vi "Core Import Validation.vi"(6 "Slot Number":u32, 7 "File to Import":path, 8 "error in (no error)":errorcluster, 9 "Endpoint Configurations":T1[](array[typedef]), 10 "Switch Properties":T3, 11 "SLSC Switch Import Unit Tests in":refnum<class "SLSC Switch Import Unit Tests.lvclass">) -> (0 "error out":errorcluster, 3 "SLSC Switch Import Unit Tests out":refnum<class "SLSC Switch Import Unit Tests.lvclass">)   [LabVIEW 2017, in "SLSC Switch Import Unit Tests.lvclass"]
uses:
  SLSC Switch Import Unit Tests.lvclass
  Scripting/Properties/SLSC Switch All Properties.ctl
  Shared/Endpoint Configuration Cluster.ctl
  Shared/Endpoint Configuration Enum.ctl
  SLSC Switch Import Unit Tests.lvclass/SLSC Switch Import Unit Tests.ctl
  <userlib>/_OpenG.lib/file/file.llb/Append Path to Root if Relative - Scalar__ogtk.vi
  <vilib>/NI Veristand/Custom Device API/Get Item Property (I32).vi
  Scripting/SLSC Switch Scripting.lvlib
  niveristand-custom-device-testing-tools/VeriStandTestUtilities/VeriStandTestUtilities.lvlib
  <vilib>/NI VeriStand/Custom Device API/Custom Device API.lvlib
  Shared/Routing and Faulting Hardware API/Routing and Faulting Hardware API.lvlib
  Shared/SLSC Switch Shared.lvlib
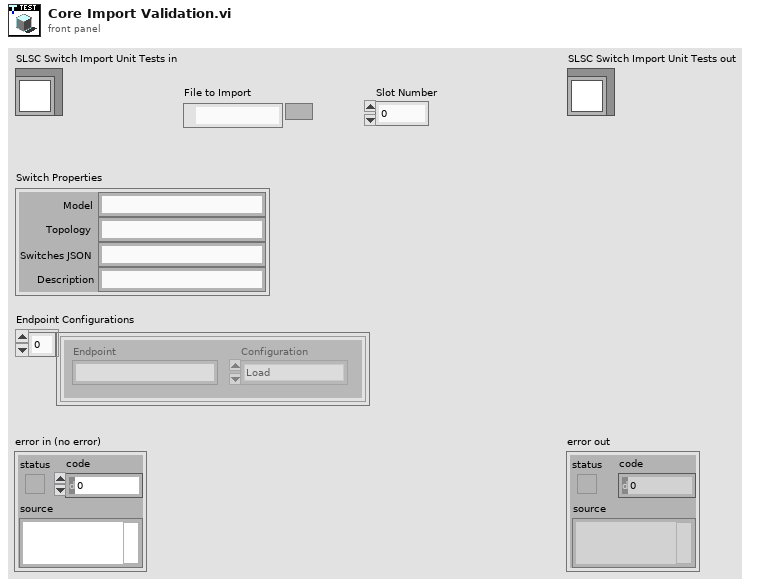
[diagram p1: front panel]
types:
  T1 = typedef "SLSC Switch Shared.lvlib/Endpoint Configuration Cluster.ctl" = cluster{"Endpoint":string, "Configuration":T2}
  T2 = typedef "SLSC Switch Shared.lvlib/Endpoint Configuration Enum.ctl" = enum16{"Load", "Source", "Configuration"}
  T3 = typedef "SLSC Switch Scripting.lvlib/SLSC Switch All Properties.ctl" = cluster{"Model":string, "Topology":string, "Switches JSON":string, "Description":string}
  T4 = typedef "Custom Device API.lvlib/Custom Device Item Ref.ctl" = u64
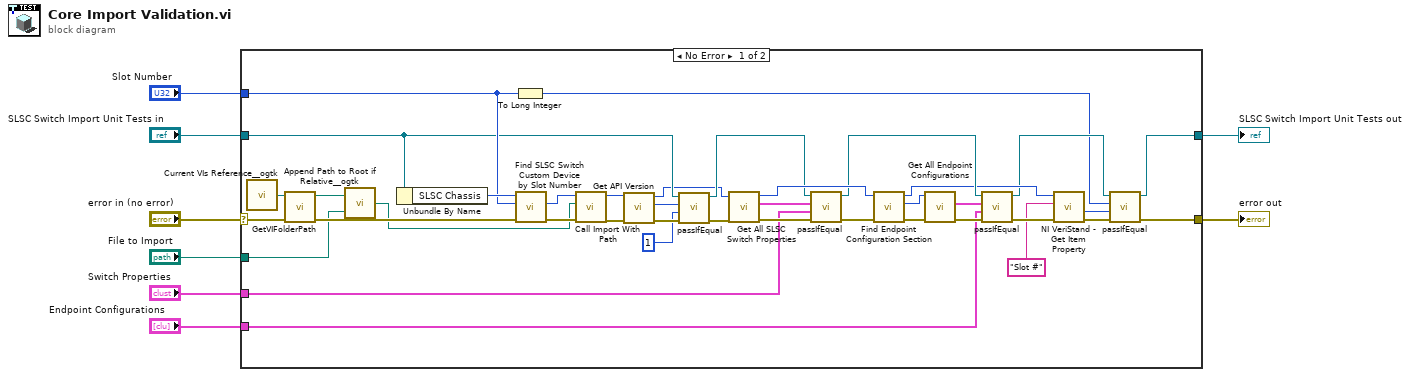
[diagram p0: block diagram]
diagram:
  n1 = case shown="No Error" "error in (no error)" {
    selector: "error in (no error)" -> [w19 w49]
    tunnel: [w18 w49] -> w7
    tunnel: [w20 w48] -> w5
    tunnel: "SLSC Switch Import Unit Tests in" -> [w11 w48]
    tunnel: "File to Import" -> [w24 _]
    tunnel: "Slot Number" -> [w23 _]
    tunnel: "Switch Properties" -> [w22 _]
    tunnel: "Endpoint Configurations" -> [w21 _]
    frame No Error {
      n2 = call <userlib>:"Current VIs Reference__ogtk.vi"() -> ("Current VI's reference"=w44:refnum<vi>)  [unwired: 5 in]
      n3 = call "GetVIFolderPath.vi"("error in (no error)"=w19, "VI Reference in"=w44) -> ("error out"=w42:errorcluster, "VI Folder Path out"=w43:path)  [unwired: 8 in]
      n4 = call-poly <userlib>:"Append Path to Root if Relative__ogtk.vi"("Absolute or Relative Path"=w24, "Root Path"=w43) -> ("Absolute or Appended Path"=w41:path)
      n5 = Unbundle By Name(w11) -> ("SLSC Chassis"=w47:u64)
      n6 = To Long Integer(number=w23) -> (32bit integer=w26:i32)
      n7 = call "Find SLSC Switch Custom Device by Slot Number.vi"("error in (no error)"=w42, "slot number"=w23, "SLSC Chassis Ref"=w47) -> ("error out"=w46:errorcluster, "SLSC Switch Custom Device Ref"=w45:T4)  [unwired: 6 in, 1 out]
      n8 = call "Call Import With Path.vi"("error in (no error)"=w46, "Path"=w41, "Node Ptr"=w45) -> ("error out"=w16:errorcluster, "Node Ptr out"=w17:u64)  [unwired: 7 in]
      n9 = call "Get API Version.vi"("error in (no error)"=w16, "Hardware Ref in"=w17) -> ("error out"=w15:errorcluster, "API version"=w13:u32, "Hardware Ref out"=w9:T4)  [unwired: 6 in, 1 out]
      n10 = call-dynamic "passIfEqual.vi"("error in (no error)"=w15, "y"=u32 1 ("API version"), "x"=w13, "TestCase in"=w11) -> ("error out"=w14:errorcluster, "TestCase out"=w10:refnum<class "SLSC Switch Import Unit Tests.lvclass">)  [unwired: 6 in]
      n11 = call "Get All SLSC Switch Properties.vi"("error in (no error)"=w14, "SLSC Switch Custom Device Ref in"=w9) -> ("error out"=w40:errorcluster, "SLSC Switch All Properties"=w39:T3, "SLSC Switch Custom Device Ref out"=w36:T4)  [unwired: 7 in]
      n12 = call-dynamic "passIfEqual.vi"("error in (no error)"=w40, "y"=w22, "x"=w39, "TestCase in"=w10) -> ("error out"=w38:errorcluster, "TestCase out"=w34:refnum<class "SLSC Switch Import Unit Tests.lvclass">)  [unwired: 6 in]
      n13 = call "Find Endpoint Configuration Section.vi"("error in (no error)"=w38, "SLSC Switch Custom Device Ref in"=w36) -> ("error out"=w37:errorcluster, "Endpoint Config Section Ref"=w25:T4, "SLSC Switch Custom Device Ref out"=w30:T4)  [unwired: 7 in]
      n14 = call "Get All Endpoint Configurations.vi"("error in (no error)"=w37, "Endpoint Configuration Section Ref in"=w25) -> ("error out"=w35:errorcluster, "All Endpoint Configurations"=w33:T1[])  [unwired: 7 in, 1 out]
      n15 = call-dynamic "passIfEqual.vi"("error in (no error)"=w35, "y"=w21, "x"=w33, "TestCase in"=w34) -> ("error out"=w32:errorcluster, "TestCase out"=w28:refnum<class "SLSC Switch Import Unit Tests.lvclass">)  [unwired: 6 in]
      n16 = call-poly <vilib>:"NI VeriStand - Get Item Property.vi"("error in (no error)"=w32, "Property Name"="Slot #", "Item Ref in"=w30) -> ("error out"=w29:errorcluster, "Value"=w27:i32)  [unwired: 5 in, 2 out]
      n17 = call-dynamic "passIfEqual.vi"("error in (no error)"=w29, "y"=w27, "x"=w26, "TestCase in"=w28) -> ("error out"=w18:errorcluster, "TestCase out"=w20:refnum<class "SLSC Switch Import Unit Tests.lvclass">)  [unwired: 6 in]
    }
    frame Error {
    }
  }
  "error out" <- w7
  "SLSC Switch Import Unit Tests out" <- w5
